vi "Select Instrument Type.vi"(11 "Numeric":i32) -> (3 "Type":string)   [LabVIEW 2019, in "Control Experiment.lvclass"]
uses:
  Control Experiment.lvclass
  Typedefs/Instrument Types--combo.ctl
panel:
  in  "Instrument Types":T1="Temperature"
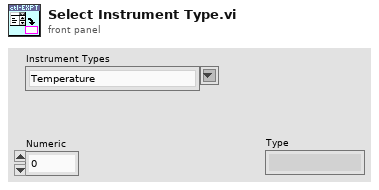
[diagram p1: front panel]
types:
  T1 = typedef "Control Experiment.lvclass/Instrument Types--combo.ctl" = string
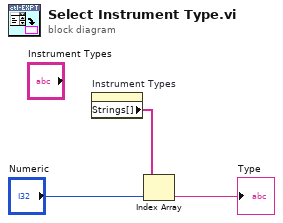
[diagram p0: block diagram]
diagram:
  n1 = property on="Instrument Types" class="CmbBox (strict)"() -> ("Strings[]"=w3:string[])  [unwired: 2 in, 2 out]
  n2 = Index Array(array=w3, index="Numeric") -> (element=→"Type":string)
